vi "Read Path.vi"(8 "error in (no error)":errorcluster, 11 "ElectrometerError in":refnum<class "ElectrometerError.lvclass">) -> (0 "error out":errorcluster, 2 "Path":path, 3 "ElectrometerError out":refnum<class "ElectrometerError.lvclass">)   [LabVIEW 2016, in "ElectrometerError.lvclass"]
uses:
  ElectrometerError.lvclass
  ElectrometerError.lvclass/ElectrometerError.ctl
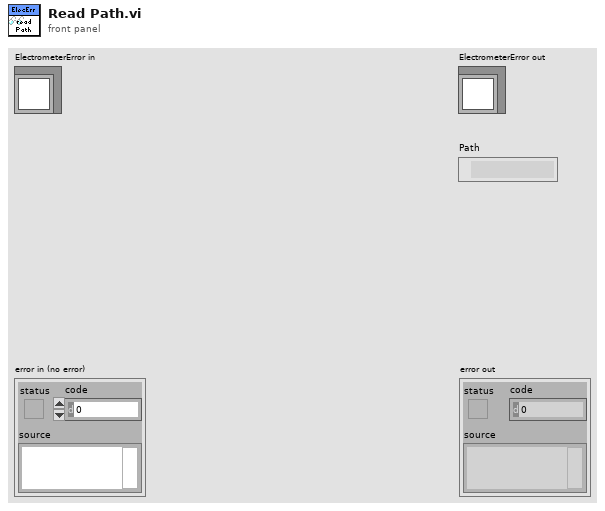
[diagram p1: front panel]
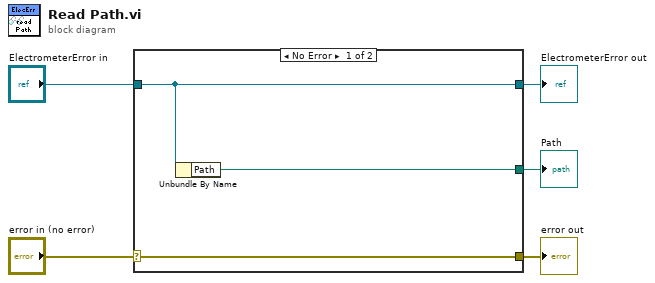
[diagram p0: block diagram]
diagram:
  n1 = case shown="No Error" "error in (no error)" {
    selector: "error in (no error)" -> [w8 w9]
    tunnel: [w8 w9] -> w4
    tunnel: [w7 w10] -> w2
    tunnel: "ElectrometerError in" -> [w7 w10]
    tunnel: [w6 _] -> w1
    frame No Error {
      n2 = Unbundle By Name(w7) -> ("Path"=w6:path)
    }
    frame Error {
    }
  }
  "error out" <- w4
  "ElectrometerError out" <- w2
  "Path" <- w1
